vi "Function 2.vi"(8 "error in (no error)":errorcluster, 11 "Data Cluster":T1={"Vesta Data Output"={"Temp_W_Raw_U"=0, "Temp_W_Raw_L"=0, "Temperature Water (F)"=0.0, "Temperature Water Compensated (F)"=0.0, "Temperature Ambient (F)"=0.0, "Setpoint Location (F)"=0.0, "Heat Request"="", "Fault Ram"="", "PWM DCDC Value"=0, "Pilot Voltage (mV)"=0.0, "Setpoint Actual (F)"=0.0, "Differential Actual (F)"=0.0, "Setpoint User (F)"=0.0, "Differential User (F)"=0.0, "Termperature FIltered -TCO (F)"=0.0, "Temp_C_Raw_1 - Sensor Voltage"="", "Temp_C_Raw_2 - Sensor Voltage"="", "Chamber Sensor Temperature (F)"=0.0, "LDO Base Temperature (F)"=0.0, "LDO Timer (sec)"=0, "Disabled (0)"=FALSE, "Warming (1)"=FALSE, "Heating (2)"=FALSE, "Cooling Data Write (3)"=FALSE, "Cooling (4)"=FALSE, "Data Read (5)"=FALSE, "N/A"=FALSE, "Temperature Trip (7)"=FALSE, "Burner"=FALSE}, "VestaTemperature"={"Water Heater Temp (°F)"=135, "Differential  (°F)"=10.0}, "Timer Application Data"={"Duty Cycle"={"Burner ON Time (Seconds)"=60.0, "Burner OFF Time (Seconds)"=60.0, "Main Burner Flag"=FALSE, "Burner Power Mode"=0}}, "Data Array"=[], "MW Output"={"TC1-Channel 021"=0.0, "TC2-Channel 022"=0.0, "TC3-Channel 023"=0.0, "TC4-Channel 024"=0.0, "TC5-Channel 025"=0.0, "TC6-Channel 026"=0.0, "TC7-Channel 017"=0.0, "TC8-Channel 028"=0.0, "TC9-Channel 029"=0.0, "TC10-Channel 030"=0.0, "TC Tree Average"=0.0, "TC DWN- Channel 027"=0.0, "RTDin-Channel 031"=0.0, "RTDout-Channel 032"=0.0, "RTDamb-Channel 033"=0.0, "PSI1-Channel 011"=0.0, "PSI2-Channel 012"=0.0, "PSI3-Channel 013"=0.0, "PSI4-Channel 014"=0.0, "UE State-Channel 015"=0.0, "LE State-Channel 016"=0.0, "Module 4 Relay Status Output"={"INTELLIFAUCET TEMP(T)/FLOW(F) (CH 041)"=FALSE, "INTELLIFAUCET READY (CH 042)"=FALSE, "INTELLIFAUCET START (CH 043)"=FALSE, "INTELLIFAUCET STOP (CH 044)"=FALSE, "MAIN POWER RELAY (CH 047)"=FALSE, "NOT USED (CH 045)"=FALSE, "NOT USED (CH 046)"=FALSE, "PURGE VALVE RELAY (CH 048)"=FALSE, "OUTLET VALVE RELAY (CH 049)"=FALSE, "INLET VALVE RELAY (CH 050)"=FALSE, "Intellifaucet (% Open)"=0.0, "Proportioning Valve (%Open)"=0.0, "Intellifaucet Temp Setpoint (F)"=0.0}}} {"VestaTemperature"."Water Heater Temp (°F)" min=32 max=203}) -> (0 "error out":errorcluster, 3 "Data Cluster Out":T1={"Vesta Data Output"={"Temp_W_Raw_U"=0, "Temp_W_Raw_L"=0, "Temperature Water (F)"=0.0, "Temperature Water Compensated (F)"=0.0, "Temperature Ambient (F)"=0.0, "Setpoint Location (F)"=0.0, "Heat Request"="", "Fault Ram"="", "PWM DCDC Value"=0, "Pilot Voltage (mV)"=0.0, "Setpoint Actual (F)"=0.0, "Differential Actual (F)"=0.0, "Setpoint User (F)"=0.0, "Differential User (F)"=0.0, "Termperature FIltered -TCO (F)"=0.0, "Temp_C_Raw_1 - Sensor Voltage"="", "Temp_C_Raw_2 - Sensor Voltage"="", "Chamber Sensor Temperature (F)"=0.0, "LDO Base Temperature (F)"=0.0, "LDO Timer (sec)"=0, "Disabled (0)"=FALSE, "Warming (1)"=FALSE, "Heating (2)"=FALSE, "Cooling Data Write (3)"=FALSE, "Cooling (4)"=FALSE, "Data Read (5)"=FALSE, "N/A"=FALSE, "Temperature Trip (7)"=FALSE, "Burner"=FALSE}, "VestaTemperature"={"Water Heater Temp (°F)"=135, "Differential  (°F)"=10.0}, "Timer Application Data"={"Duty Cycle"={"Burner ON Time (Seconds)"=60.0, "Burner OFF Time (Seconds)"=60.0, "Main Burner Flag"=FALSE, "Burner Power Mode"=0}}, "Data Array"=[], "MW Output"={"TC1-Channel 021"=0.0, "TC2-Channel 022"=0.0, "TC3-Channel 023"=0.0, "TC4-Channel 024"=0.0, "TC5-Channel 025"=0.0, "TC6-Channel 026"=0.0, "TC7-Channel 017"=0.0, "TC8-Channel 028"=0.0, "TC9-Channel 029"=0.0, "TC10-Channel 030"=0.0, "TC Tree Average"=0.0, "TC DWN- Channel 027"=0.0, "RTDin-Channel 031"=0.0, "RTDout-Channel 032"=0.0, "RTDamb-Channel 033"=0.0, "PSI1-Channel 011"=0.0, "PSI2-Channel 012"=0.0, "PSI3-Channel 013"=0.0, "PSI4-Channel 014"=0.0, "UE State-Channel 015"=0.0, "LE State-Channel 016"=0.0, "Module 4 Relay Status Output"={"INTELLIFAUCET TEMP(T)/FLOW(F) (CH 041)"=FALSE, "INTELLIFAUCET READY (CH 042)"=FALSE, "INTELLIFAUCET START (CH 043)"=FALSE, "INTELLIFAUCET STOP (CH 044)"=FALSE, "MAIN POWER RELAY (CH 047)"=FALSE, "NOT USED (CH 045)"=FALSE, "NOT USED (CH 046)"=FALSE, "PURGE VALVE RELAY (CH 048)"=FALSE, "OUTLET VALVE RELAY (CH 049)"=FALSE, "INLET VALVE RELAY (CH 050)"=FALSE, "Intellifaucet (% Open)"=0.0, "Proportioning Valve (%Open)"=0.0, "Intellifaucet Temp Setpoint (F)"=0.0}}} {"VestaTemperature"."Water Heater Temp (°F)" min=32 max=203}, 4 "Send_Vesta_Message":u8, 6 "Send_Timer_Message":u8)   [LabVIEW 2023]
uses:
  controls/UI Data.ctl
  Drivers/Resideo Gas Valve/Type Definitions/Vesta Info.ctl
  Drivers/Resideo Gas Valve/Type Definitions/Temperature Control.ctl
  controls/Timer Application Cluster.ctl
  controls/Burner Duty Cycle.ctl
  Hybrid Water Heater/Type Definitions/HEWH MW100 Data Cluster.ctl
  Hybrid Water Heater/Custom Instrument Control/MW100/Type Definitions/HEWH Module 4 Relay Status.ctl
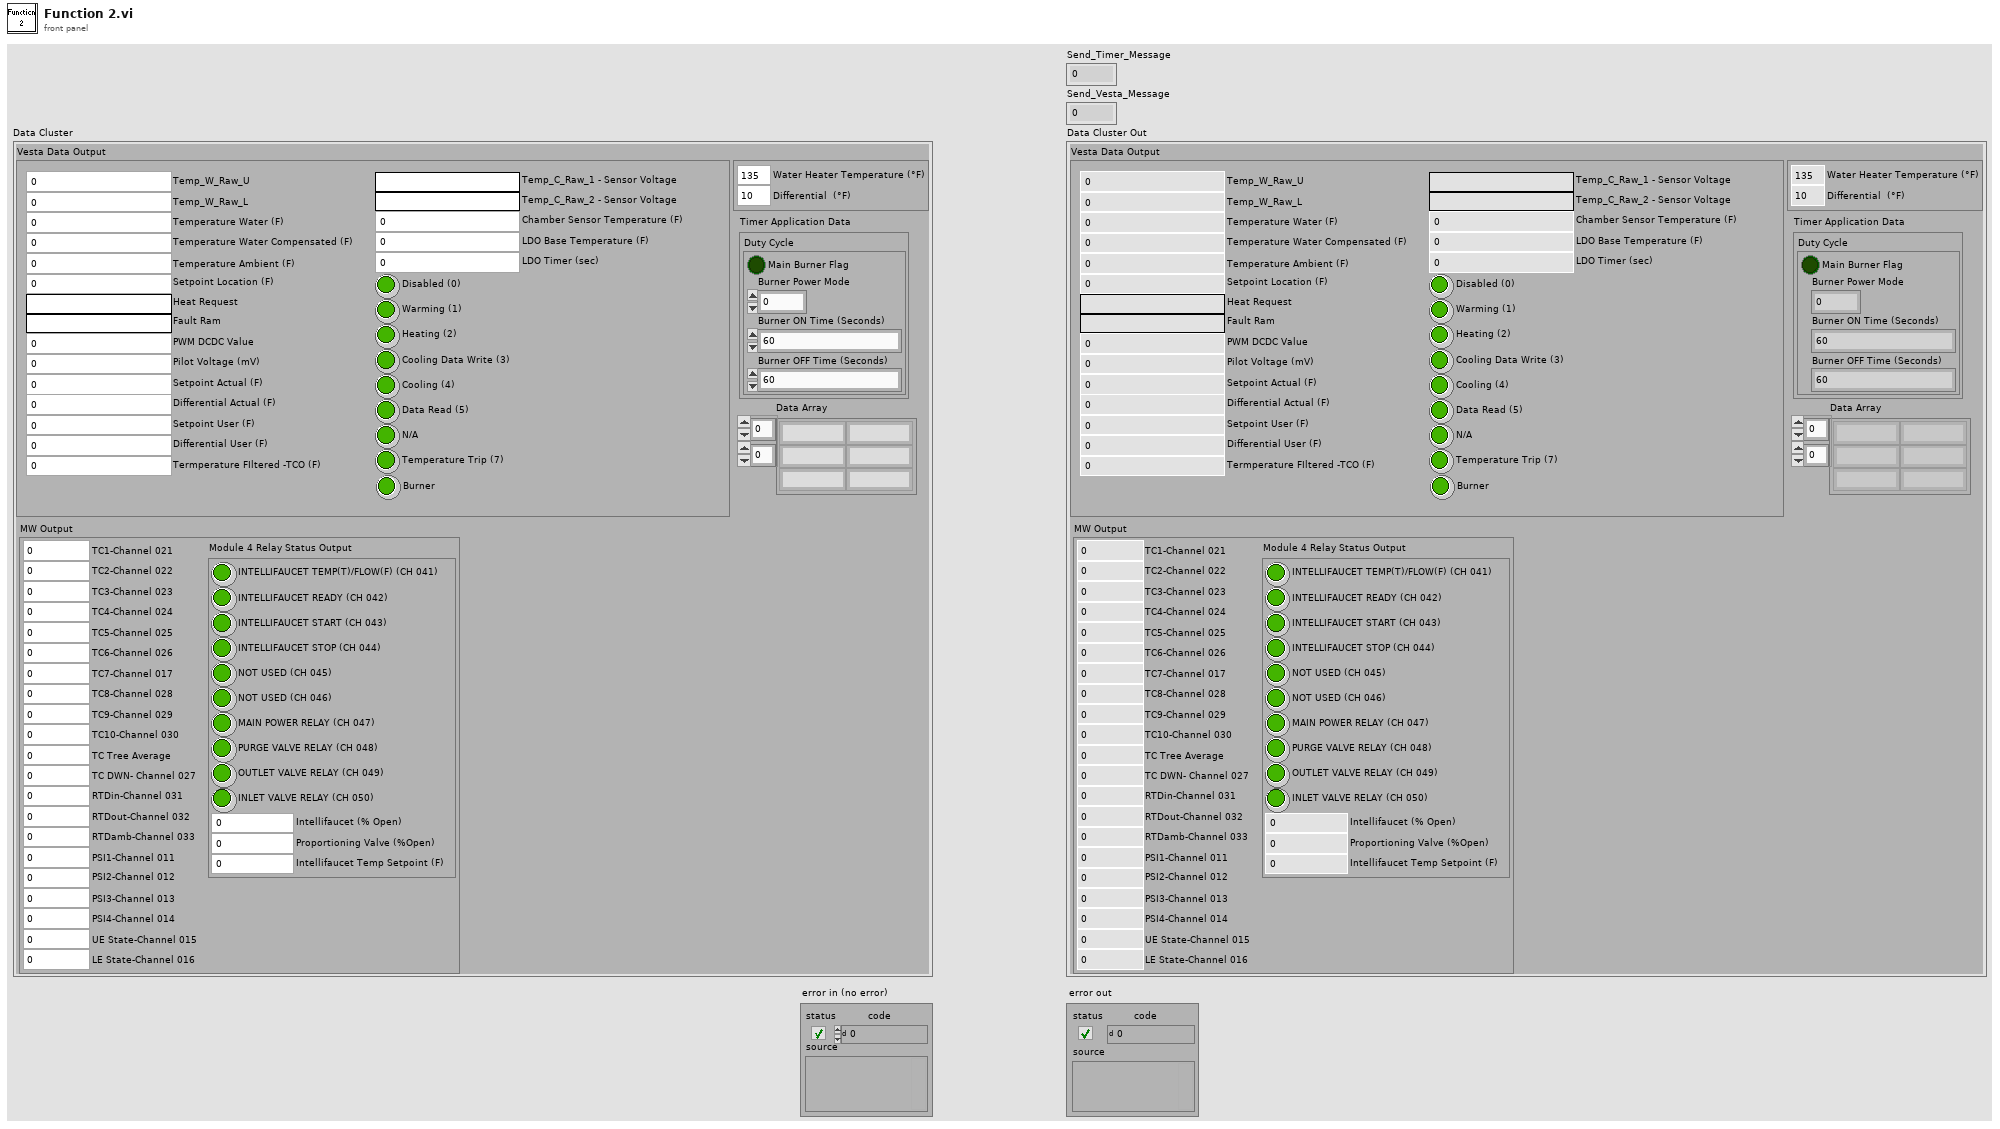
[diagram p1: front panel]
types:
  T1 = typedef "UI Data.ctl" = cluster{"Vesta Data Output":T2, "VestaTemperature":T3, "Timer Application Data":T4, "Data Array":string[][], "MW Output":T6}
  T2 = typedef "Vesta Info.ctl" = cluster{"Temp_W_Raw_U":u16, "Temp_W_Raw_L":u16, "Temperature Water (F)":dbl, "Temperature Water Compensated (F)":dbl, "Temperature Ambient (F)":dbl, "Setpoint Location (F)":dbl, "Heat Request":string, "Fault Ram":string, "PWM DCDC Value":u16, "Pilot Voltage (mV)":dbl, "Setpoint Actual (F)":dbl, "Differential Actual (F)":dbl, "Setpoint User (F)":dbl, "Differential User (F)":dbl, "Termperature FIltered -TCO (F)":dbl, "Temp_C_Raw_1 - Sensor Voltage":string, "Temp_C_Raw_2 - Sensor Voltage":string, "Chamber Sensor Temperature (F)":dbl, "LDO Base Temperature (F)":dbl, "LDO Timer (sec)":i16, "Disabled (0)":bool, "Warming (1)":bool, "Heating (2)":bool, "Cooling Data Write (3)":bool, "Cooling (4)":bool, "Data Read (5)":bool, "N/A":bool, "Temperature Trip (7)":bool, "Burner":bool}
  T3 = typedef "Temperature Control.ctl" = cluster{"Water Heater Temp (°F)":u16, "Differential  (°F)":dbl}
  T4 = typedef "Timer Application Cluster.ctl" = cluster{"Duty Cycle":T5}
  T5 = typedef "Burner Duty Cycle.ctl" = cluster{"Burner ON Time (Seconds)":dbl, "Burner OFF Time (Seconds)":dbl, "Main Burner Flag":bool, "Burner Power Mode":u8}
  T6 = typedef "HEWH MW100 Data Cluster.ctl" = cluster{"TC1-Channel 021":dbl, "TC2-Channel 022":dbl, "TC3-Channel 023":dbl, "TC4-Channel 024":dbl, "TC5-Channel 025":dbl, "TC6-Channel 026":dbl, "TC7-Channel 017":dbl, "TC8-Channel 028":dbl, "TC9-Channel 029":dbl, "TC10-Channel 030":dbl, "TC Tree Average":dbl, "TC DWN- Channel 027":dbl, "RTDin-Channel 031":dbl, "RTDout-Channel 032":dbl, "RTDamb-Channel 033":dbl, "PSI1-Channel 011":dbl, "PSI2-Channel 012":dbl, "PSI3-Channel 013":dbl, "PSI4-Channel 014":dbl, "UE State-Channel 015":dbl, "LE State-Channel 016":dbl, "Module 4 Relay Status Output":T7}
  T7 = typedef "HEWH Module 4 Relay Status.ctl" = cluster{"INTELLIFAUCET TEMP(T)/FLOW(F) (CH 041)":bool, "INTELLIFAUCET READY (CH 042)":bool, "INTELLIFAUCET START (CH 043)":bool, "INTELLIFAUCET STOP (CH 044)":bool, "MAIN POWER RELAY (CH 047)":bool, "NOT USED (CH 045)":bool, "NOT USED (CH 046)":bool, "PURGE VALVE RELAY (CH 048)":bool, "OUTLET VALVE RELAY (CH 049)":bool, "INLET VALVE RELAY (CH 050)":bool, "Intellifaucet (% Open)":dbl, "Proportioning Valve (%Open)":dbl, "Intellifaucet Temp Setpoint (F)":dbl}
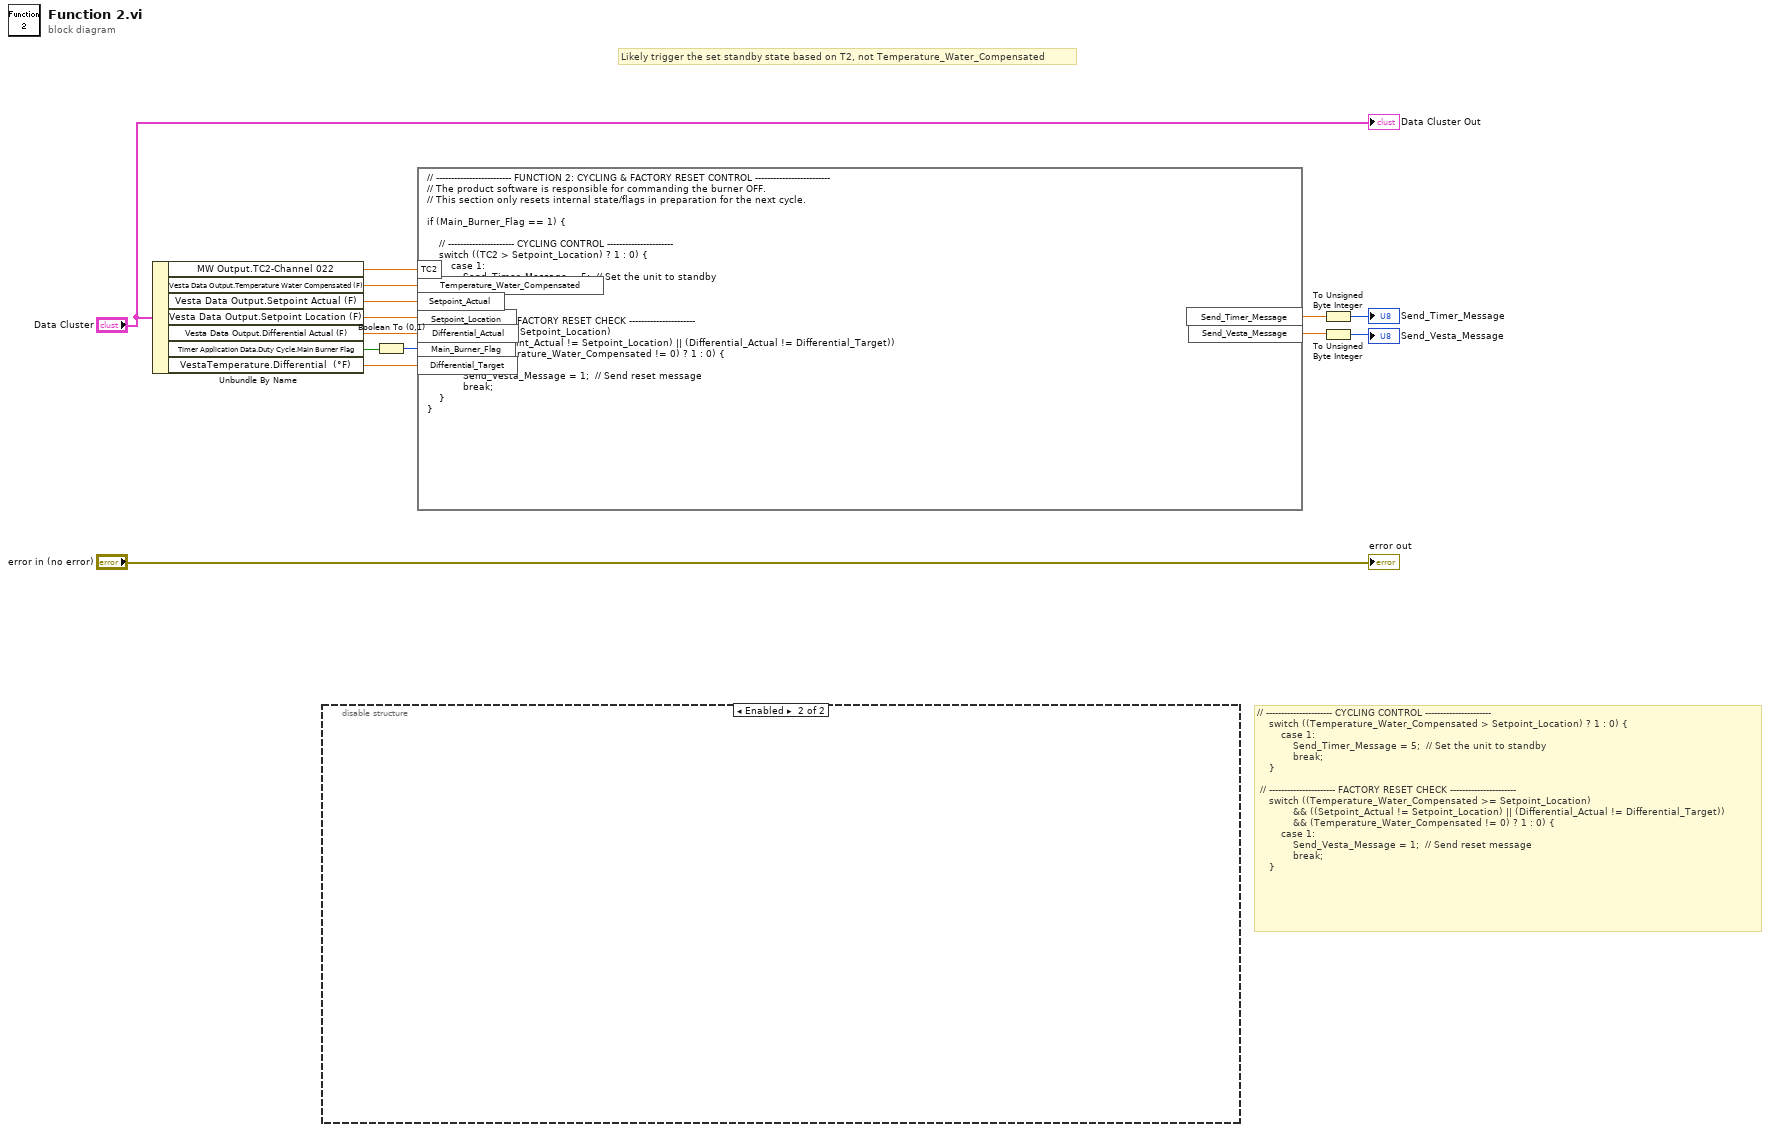
[diagram p0: block diagram]
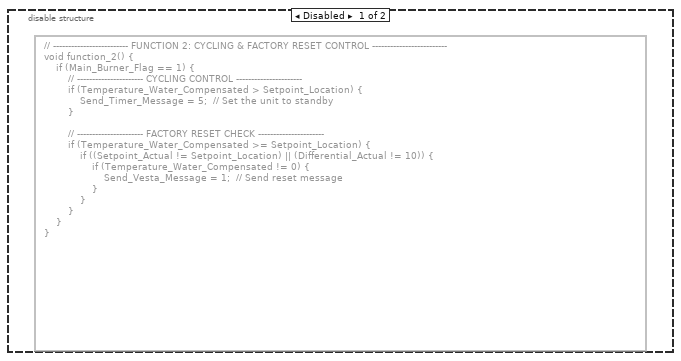
[diagram p2: hidden frame]
diagram:
  # "// ---------------------- CYCLING CONTROL ----------------------\n    switch ((Temperature_Water_Compensated > Setpoint_Location) ? 1 : 0) {\n        case 1:\n            Send_Timer_Message = 5;  // Set the unit to standby\n            break;\n    }\n\n // ---------------------- FACTORY RESET CHECK ----------------------\n    switch ((Temperature_Water_Compensated >= Setpoint_Location) \n            && ((Setpoint_Actual != Setpoint_Location) || (Differential_Actual != Differential_Target)) \n            && (Temperature_Water_Compensated != 0) ? 1 : 0) {\n        case 1:\n            Send_Vesta_Message = 1;  // Send reset message\n            break;\n    }"
  # "Likely trigger the set standby state based on T2, not Temperature_Water_Compensated"
  n1 = Unbundle By Name("Data Cluster") -> ("MW Output.TC2-Channel 022"=w1:dbl, "Vesta Data Output.Temperature Water Compensated (F)"=w8:dbl, "Vesta Data Output.Setpoint Actual (F)"=w6:dbl, "Vesta Data Output.Setpoint Location (F)"=w7:dbl, "Vesta Data Output.Differential Actual (F)"=w5:dbl, "Timer Application Data.Duty Cycle.Main Burner Flag"=w14:bool, "VestaTemperature.Differential  (°F)"=w2:dbl)
  n2 = disable-structure shown="Enabled" {
    frame Disabled {
      n3 = formula code="// ------------------------- FUNCTION 2: CYCLING & FACTORY RESET CONTROL -------------------------\nvoid function_2() {\n    if (Main_Burner_Flag == 1) {\n        // ---------------------- CYCLING CONTROL ----------------------\n        if (Temperature_Water_Compensated > Setpoint_Location) {\n            Send_Timer_Message = 5;  // Set the unit to standby\n        } \n\n        // ---------------------- FACTORY RESET CHECK ----------------------\n        if (Temperature_Water_Compensated >= Setpoint_Location) {  \n            if ((Setpoint_Actual != Setpoint_Location) || (Differential_Actual != 10)) {  \n                if (Temperature_Water_Compensated != 0) {  \n                    Send_Vesta_Message = 1;  // Send reset message\n                }\n            }\n        }\n    }\n}"() -> ()
    }
    frame Enabled {
    }
  }
  n4 = Boolean To (0,1)(Boolean=w14) -> (0, 1=w4:i16)
  n5 = formula code="// ------------------------- FUNCTION 2: CYCLING & FACTORY RESET CONTROL -------------------------\n// The product software is responsible for commanding the burner OFF.\n// This section only resets internal state/flags in preparation for the next cycle.\n\nif (Main_Burner_Flag == 1) {\n\n    // ---------------------- CYCLING CONTROL ----------------------\n    switch ((TC2 > Setpoint_Location) ? 1 : 0) {\n        case 1:\n            Send_Timer_Message = 5;  // Set the unit to standby\n            break;\n    }\n\n    // ---------------------- FACTORY RESET CHECK ----------------------\n    switch ((TC2 >= Setpoint_Location) \n            && ((Setpoint_Actual != Setpoint_Location) || (Differential_Actual != Differential_Target)) \n            && (Temperature_Water_Compensated != 0) ? 1 : 0) {\n        case 1:\n            Send_Vesta_Message = 1;  // Send reset message\n            break;\n    }\n}"("Main_Burner_Flag"=w4, "Temperature_Water_Compensated"=w8, "Setpoint_Location"=w7, "Setpoint_Actual"=w6, "Differential_Actual"=w5, "Differential_Target"=w2, "TC2"=w1) -> ("Send_Vesta_Message"=w9:dbl, "Send_Timer_Message"=w10:dbl)
  n6 = To Unsigned Byte Integer(number=w10) -> (unsigned 8bit integer=→"Send_Timer_Message":u8)
  n7 = To Unsigned Byte Integer(number=w9) -> (unsigned 8bit integer=→"Send_Vesta_Message":u8)
  "Data Cluster Out" <- "Data Cluster"
  "error out" <- "error in (no error)"
